vi "UI.vi"() -> ()   [LabVIEW 2024, in "Scripts.lvlib"]
uses:
  Scripts.lvlib
  UI-Platform--radio.ctl
  UI-ErrorCheckingLevel--radio.ctl
  UI-Cmd--cluster.ctl
  UI-Cmd--enum.ctl
  UI-State--cluster.ctl
  UI-Refs--cluster.ctl
panel:
  out "Title":string="SDL Scripts"
  in  "ErrCheckLvl":T1 caption="Call Library Error Checking Level"
  in  "Platform":T2
  out "Progress Bar":dbl(slide) scale=0.0..10.0
  in  "Ok":bool
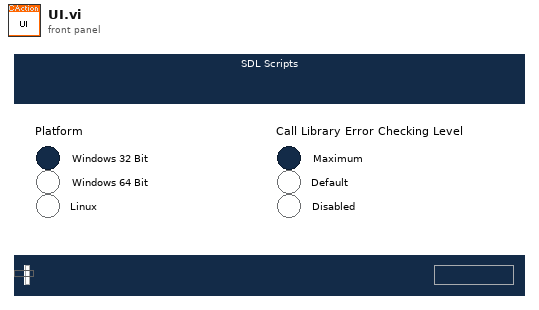
[diagram p1: front panel]
types:
  T1 = typedef "Scripts.lvlib/UI-ErrorCheckingLevel--radio.ctl" = enum32{"Maximum", "Default", "Disabled"}
  T2 = typedef "Scripts.lvlib/UI-Platform--radio.ctl" = enum32{"Windows 32 Bit", "Windows 64 Bit", "Linux"}
  T3 = typedef "Scripts.lvlib/UI-State--cluster.ctl" = cluster{"Refs":T4}
  T4 = typedef "Scripts.lvlib/UI-Refs--cluster.ctl" = cluster{"Progress Bar":refnum<vi>, "Platform":refnum<vi>}
  T5 = typedef "Scripts.lvlib/UI-Cmd--enum.ctl" = enum16{"Init", "Quit"}
  T6 = typedef "Scripts.lvlib/UI-Cmd--cluster.ctl" = cluster{"Cmd":T5, "Data":variant}
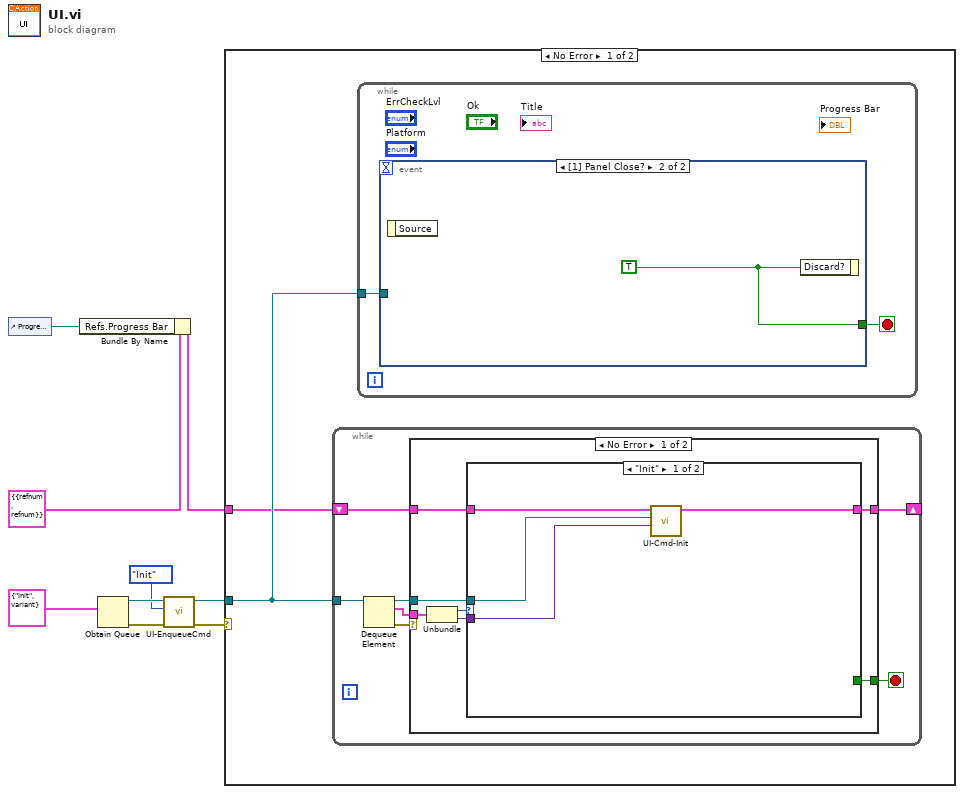
[diagram p0: block diagram]
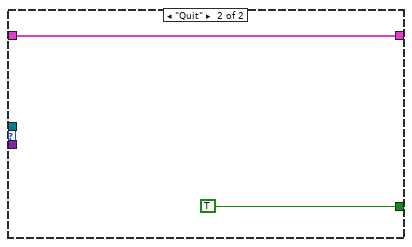
[diagram p2: hidden frame]
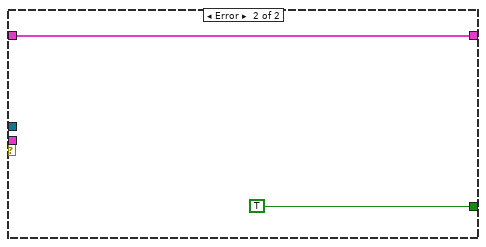
[diagram p3: hidden frame]
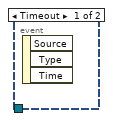
[diagram p4: hidden frame]
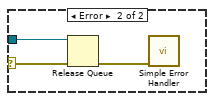
[diagram p5: hidden frame]
diagram:
  n1 = control-ref of="Progress Bar"() -> (w1:refnum<vi>)
  n2 = Bundle By Name(cluster=T3 {"Refs"={"Progress Bar"=refnum, "Platform"=refnum}} ("UI State"), "Refs.Progress Bar"=w1) -> (w2:T3)
  n3 = Obtain Queue(element data type=T6 {"Cmd"=enum."Init", "Data"=variant} ("Cmd")) -> (queue out=w8:refnum<queue>, error out=w7:errorcluster)  [unwired: 4 in, 1 out]
  n4 = call "UI-EnqueueCmd.vi"("error in (no error)"=w7, "Cmd"=UI-Cmd--enum."Init", "Queue In"=w8) -> ("error out"=w6:errorcluster, "Queue Out"=w5:refnum<queue>)  [unwired: 7 in]
  n5 = case shown="No Error" w6 {
    selector: w6 -> [_ w38]
    tunnel: w5 -> [w11 w39]
    tunnel: w2 -> [w10 _]
    frame No Error {
      n6 = while {
        tunnel: w11 -> [w18]
        shift-right: [w13] -> _
        shift-left: w10 -> [w14]
        stop <- w16 stop-if-true
        n7 = Dequeue Element(queue=w18) -> (queue out=w12:refnum<queue>, element=w17:T6, error out=w15:errorcluster)  [unwired: 2 in, 1 out]
        n8 = case shown="No Error" w15 {
          tunnel: w17 -> [w25 _]
          tunnel: [w22 TRUE] -> w16
          tunnel: w14 -> [w21 w32]
          tunnel: [w20 w32] -> w13
          tunnel: w12 -> [w19 _]
          frame No Error {
            n9 = Unbundle(w25) -> ("Cmd"=w24:T5, "Data"=w23:variant)
            n10 = case shown="\"Init\"" w24 {
              tunnel: w23 -> [w26 _]
              tunnel: [_ TRUE] -> w22
              tunnel: w21 -> [w29 w30]
              tunnel: [w28 w30] -> w20
              tunnel: w19 -> [w27 _]
              frame "Init" {
                n11 = call "UI-Cmd-Init.vi"("Data"=w26, "Queue"=w27, "UI State In"=w29) -> ("UI State Out"=w28:T3)  [unwired: 7 in, 1 out]
              }
              frame "Quit" {
              }
            }
          }
          frame Error {
          }
        }
      }
      n12 = while {
        tunnel: w11 -> [w34]
        stop <- w35 stop-if-true
        n13 = event shown="[1] Panel Close?" {
          selector: _ -> [_ _]
          dyn-events: _ -> [_ _]
          timeout: _ -> [_ _]
          tunnel: [_ w36] -> w35
          tunnel: w34 -> [_ _]
          event Timeout {
            n14 = event-data() -> ()  [unwired: 1 in, 3 out]
          }
          event Panel Close? {
            w36 = TRUE ("Discard?")
            n15 = event-data() -> ()  [unwired: 1 in, 1 out]
            n16 = event-data("Discard?"=w36) -> ()  [unwired: 1 in, 1 out]
          }
        }
      }
    }
    frame Error {
      n17 = Release Queue(queue=w39, error in (no error)=w38) -> (error out=w37:errorcluster)  [unwired: 1 in, 2 out]
      n18 = call <vilib>:"Simple Error Handler.vi"("error in (no error)"=w37) -> ()  [unwired: 4 in, 5 out]
    }
  }
